vi "Recurse Pointer IDs.vi"(8 "error in (no error)":errorcluster, 9 "Type":variant, 10 "ID":string, 11 "Linked List Ref":refnum<data-value>) -> (0 "error out":errorcluster, 2 "ID out":string, 3 "Linked List Ref out":refnum<data-value>)   [LabVIEW 2019, in "Linked Lists.lvlib" / "Linked List.lvclass"]
uses:
  <vilib>/gpm_packages/@cs/linked-list/Source/Linked List/Linked List/Linked List.lvclass
  <vilib>/gpm_packages/@cs/lookup-table/Source/LookupTable/LookupTable.lvclass
  <vilib>/gpm_packages/@cs/lookup-table/Source/LookupTable/LookupTable.lvclass/LookupTable.ctl
  94271a6a-4cf1-40a4-96db-03ebfb108b5d.vi
  <vilib>/gpm_packages/@cs/lookup-table/Source/LookupTable/Read Table Reference.vi
  94271a6a-4cf1-40a4-96db-03ebfb108b5d.vi/da66b99b-f5fe-410d-a34b-146abb313f64.vi
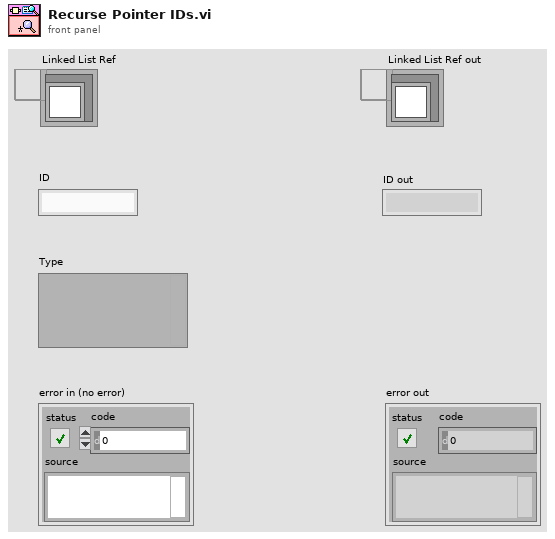
[diagram p1: front panel]
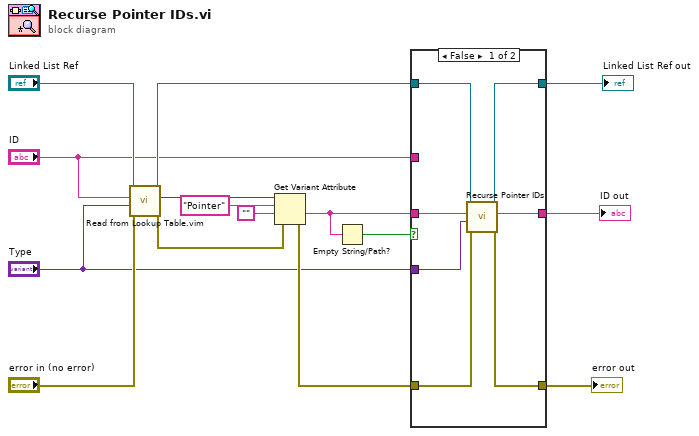
[diagram p0: block diagram]
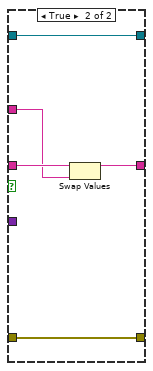
[diagram p2: hidden frame]
diagram:
  n1 = call "Read from Lookup Table.vim"("error in (no error)"="error in (no error)", "Type"="Type", "Item Name"="ID", "LookupTable Reference"="Linked List Ref") -> ("error out"=w4:errorcluster, "Value"=w1:variant, "LookupTable Reference Out"=w6:refnum<data-value>)  [unwired: 4 in, 1 out]
  n2 = Get Variant Attribute(Variant=w1, name="Pointer", default value (empty Variant)="", error in=w4) -> (value=w12:string, error out=w8:errorcluster)  [unwired: 2 out]
  n3 = Empty String/Path?(string/path=w12) -> (empty?=w10:bool)
  n4 = case shown="False" w10 {
    tunnel: [w21 w27] -> w13
    tunnel: w12 -> [w18 w25]
    tunnel: [w16 w23] -> w11
    tunnel: w6 -> [w22 w27]
    tunnel: "Type" -> [w17 _]
    tunnel: [w19 w26] -> w9
    tunnel: w8 -> [w20 w26]
    tunnel: "ID" -> [_ w24]
    frame False {
      n5 = call <vilib>:"Recurse Pointer IDs.vi"("error in (no error)"=w20, "Type"=w17, "ID"=w18, "Linked List Ref"=w22) -> ("error out"=w19:errorcluster, "ID out"=w16:string, "Linked List Ref out"=w21:refnum<data-value>)  [unwired: 5 in]
    }
    frame True {
      n6 = Swap Values(12:w25, 14:w24) -> (1:w23:string)  [unwired: 1 in, 1 out]
    }
  }
  "error out" <- w9
  "Linked List Ref out" <- w13
  "ID out" <- w11
